vi "ComunicacionVISAeste si.vi"() -> ()   [LabVIEW 2015]
doc: "This VI will continuously monitor the serial port and extract the temperature reading from the received string. This is stored in an array and displayed on the Graph. Press STOP to close the serial port and end the program.\n\nThis program is designed to work with the May 2009 version of the Arduino Temperature program which sends a header, the raw A/D value and the temperature as a float text value.\n\nSelect the appropriate COM port before running this VI. Leave the other serial port settings at their default values (9600, 8, none, 1.0, none)."
uses:
  <vilib>/Instr/_visa.llb/VISA Configure Serial Port (Instr).vi
panel:
  out "element 2":dbl
  out "element":dbl
  out "output array":dbl[](array[numeric])
  in  "VISA resource name":refnum<visa-resource-name>="COM3"
  in  "baud rate (9600)":u32=9600
  in  "data bits (8)":u16=8 min=5 max=8 step=1
  in  "stop bits (10: 1 bit)":u16(ring)=10 items=["1.0"=10, "1.5"=15, "2.0"=20]
  in  "flow control (0:none)":u16(ring) items=["None", "XON/XOFF", "RTS/CTS", "XON/XOFF & RTS/CTS", "DTR/DSR", "XON/XOFF & DTR/DSR"]
  in  "parity (0:none)":enum16{"None", "Odd", "Even", "Mark", "Space"}(ring)
  in  "stop":bool
  # "TEMP"
  # "ADC"
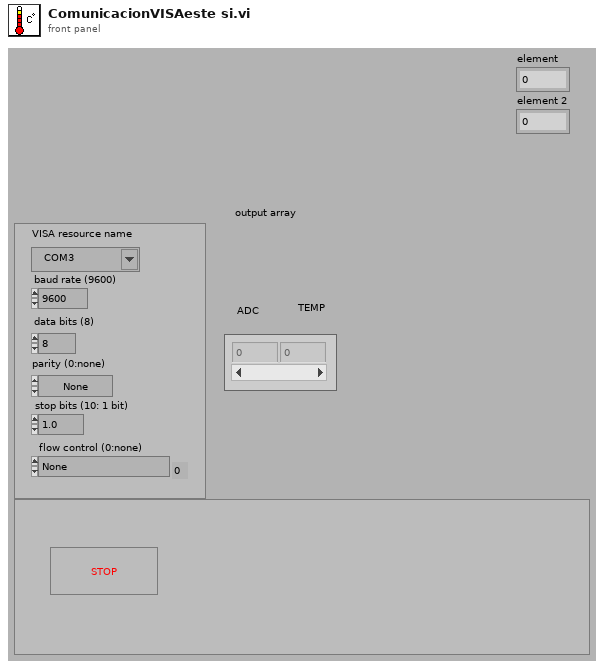
[diagram p1: front panel]
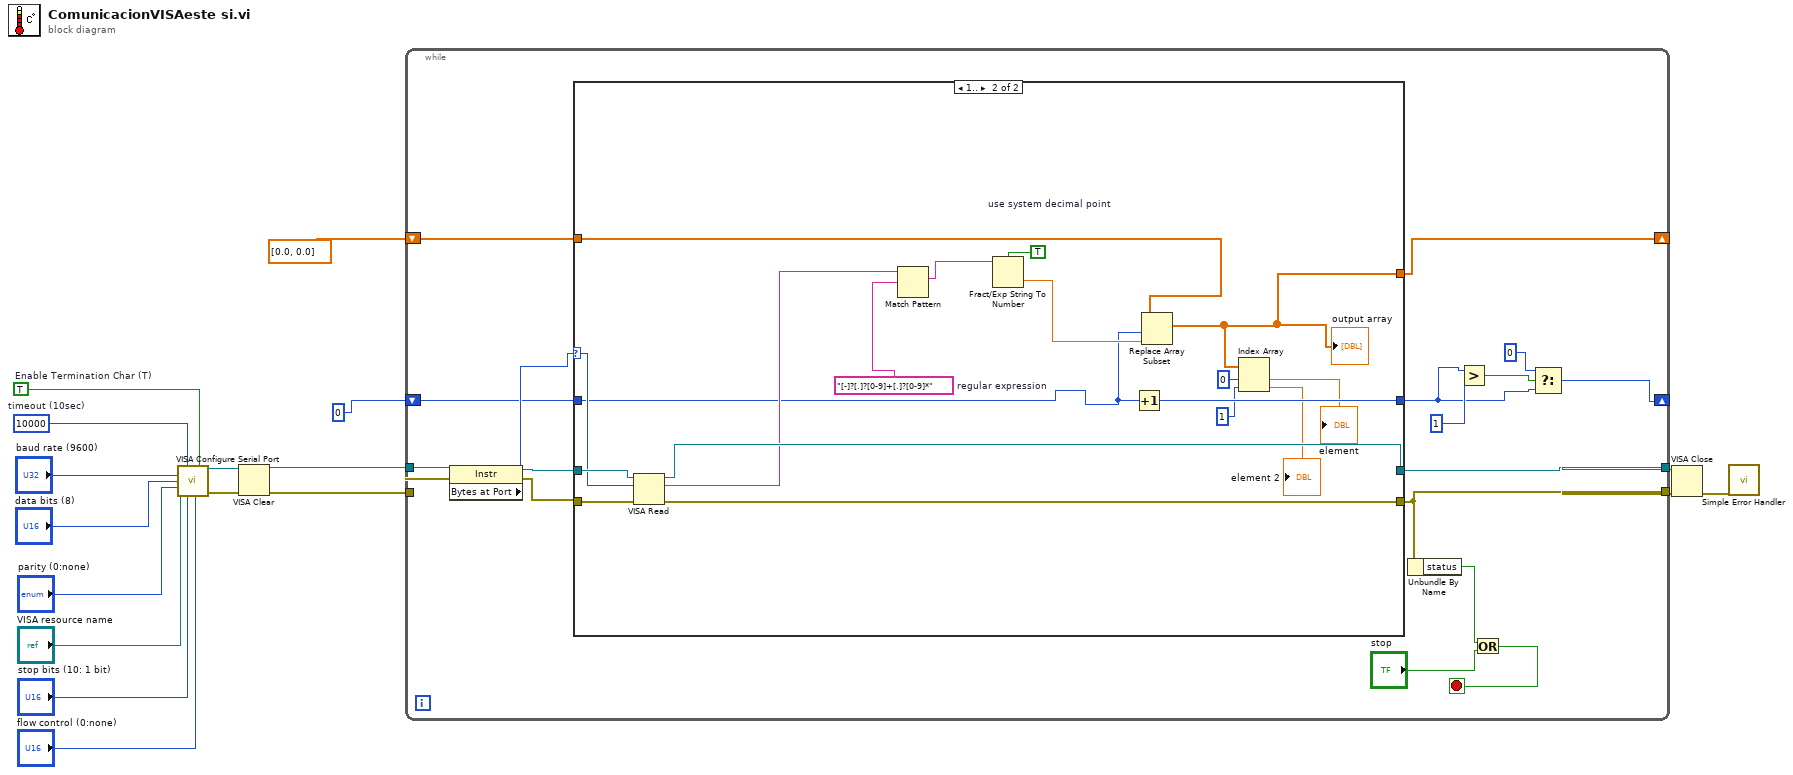
[diagram p0: block diagram]
diagram:
  w13 = TRUE  # Enable Termination Char (T)
  w14 = u32 10000  # timeout (10sec)
  n1 = call-poly "VISA Configure Serial Port"("VISA resource name"="VISA resource name", "timeout (10sec)"=w14, "Enable Termination\nChar (T)"=w13, "baud rate (9600)"="baud rate (9600)", "data bits (8)"="data bits (8)", "parity (0:none)"="parity (0:none)", "stop bits (10: 1 bit)"="stop bits (10: 1 bit)", "flow control (0:none)"="flow control (0:none)") -> ("VISA resource name out"=w11:refnum<visa-resource-name>, "error out"=w12:errorcluster)  [unwired: 6 in]
  n2 = VISA Clear(VISA resource name=w11, error in (no error)=w12) -> (VISA resource name out=w10:refnum<visa-resource-name>, error out=w3:errorcluster)
  n3 = while {
    tunnel: [w28] -> w17
    tunnel: [w30] -> w16
    tunnel: w10 -> [w32]
    tunnel: w3 -> [w31]
    shift-right: [w21] -> _
    shift-left: 0 -> [w25]
    shift-right: [w18] -> _
    shift-left: dbl[] [0.0, 0.0] -> [w23]
    stop <- w35 stop-if-true
    n4 = property class="Instr"(reference=w32, error in=w31) -> (reference out=w29:refnum<visa-resource-name>, error out=w27:errorcluster, "Bytes at Port"=w26:u32)
    n5 = case shown="1.." w26 {
      selector: w26 -> [_ w55]
      tunnel: [w39 w54] -> w30
      tunnel: w29 -> [w39 w57]
      tunnel: [w38 w53] -> w28
      tunnel: w27 -> [w38 w56]
      tunnel: [w37 w47] -> w20
      tunnel: w25 -> [w37 w46]
      tunnel: w23 -> [w36 w45]
      tunnel: [w36 w44] -> w18
      frame 0, Default {
      }
      frame 1.. {
        w52 = "[-]?[.]?[0-9]+[.]?[0-9]*"  # regular expression
        w50 = TRUE  # use system decimal point
        n6 = VISA Read(VISA resource name=w57, byte count=w55, error in (no error)=w56) -> (VISA resource name out=w54:refnum<visa-resource-name>, read buffer=w48:string, error out=w53:errorcluster)  [unwired: 1 out]
        n7 = Match Pattern(string=w48, regular expression=w52) -> (match substring=w51:string)  [unwired: 1 in, 3 out]
        n8 = Fract/Exp String To Number(use system decimal point (T)=w50, string=w51) -> (number=w49:dbl)  [unwired: 2 in, 1 out]
        n9 = Increment(x=w46) -> (x+1=w47:i32)
        n10 = Replace Array Subset(array=w45, new element=w49, index=w46) -> (w44:dbl[])
        "output array" <- w44
        n11 = Index Array(array=w44, index #1=0 ("index"), index #2=1 ("index")) -> (element #1=→"element":dbl, element #2=→"element 2":dbl)
      }
    }
    n12 = Unbundle By Name(w28) -> ("status"=w34:bool)
    n13 = Greater?(x=w20, y=1) -> (0:w22:bool)
    n14 = Or(x=w34, y="stop") -> (x .or. y?=w35:bool)
    n15 = Select(t=0, s=w22, f=w20) -> (s? t:f=w21:i32)
  }
  n16 = VISA Close(VISA resource name=w16, error in (no error)=w17) -> (error out=w15:errorcluster)
  n17 = call <vilib>:"Simple Error Handler.vi"("error in (no error)"=w15) -> ()  [unwired: 4 in, 5 out]
